vi "NI_controller_PVC.VI"(5 "Initialize":bool=TRUE, 6 "Z (mm)":dbl, 7 "Motion System":u16(ring)=3 items=["MM3000", "WMC Servo", "RRI Rot", "RRI SMAC", "Aero NI", "RRI LinInd"], 8 "error in":errorcluster, 9 "Y (mm)":dbl, 10 "X (mm)":dbl, 11 "Motion ID":T1=1 min=1 max=32 step=1) -> (0 "error out":errorcluster)   [LabVIEW 2022 SP3]
uses:
  <vilib>/Motion/FlexMotion/CustomControls/CustomControls.llb/AxisOrVectorSpace To Configure.flx
  <vilib>/Motion/FlexMotion/FunctionsVIs/StartStopMotion.llb/Start Motion (8 axes).flx
panel:
  # "X Axis"
  # "Y Axis"
  # "Z Axis"
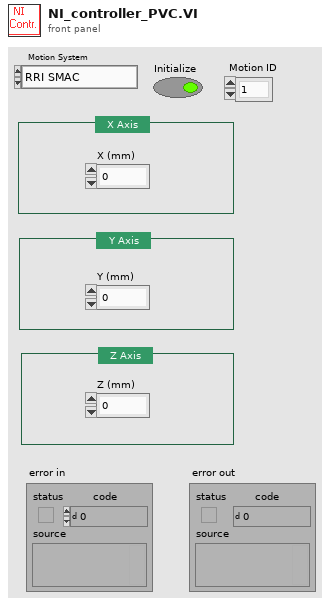
[diagram p1: front panel]
types:
  T1 = typedef "Board Id" = u8
  T2 = typedef "AxisOrVectorSpace To Configure.flx" = u16
  T3 = enum16{"Absolute Position", "Relative Position", "Velocity", "Relative to Cap Pos", "Modulus Position", "Absolute Contouring", "Relative Contouring"}
  T4 = typedef "Bd Id Out" = u8
  T5 = typedef "Resource Out (Enum).flx" = u16
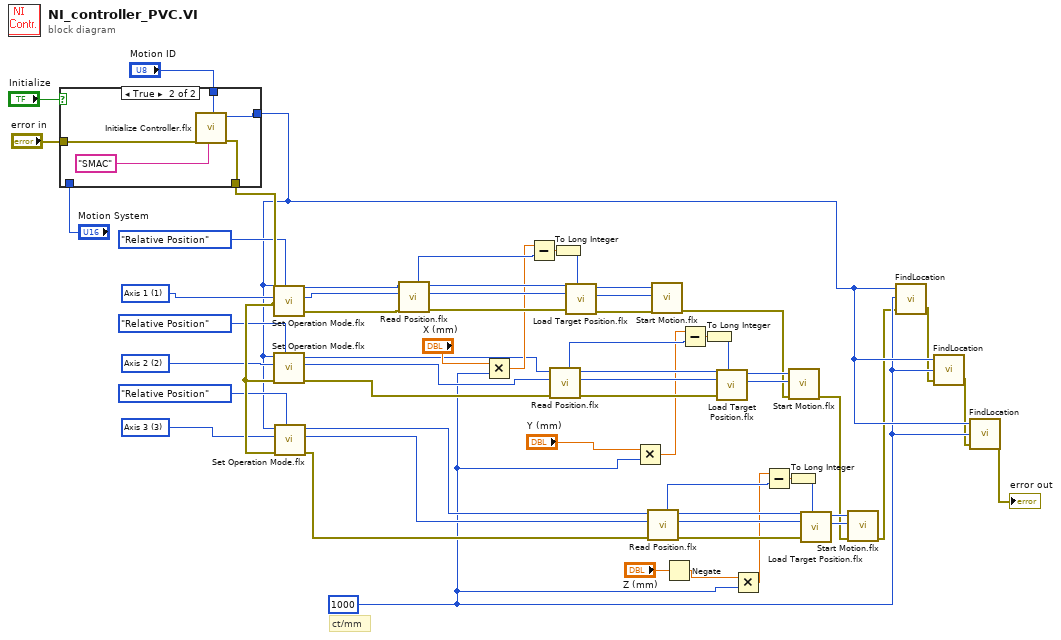
[diagram p0: block diagram]
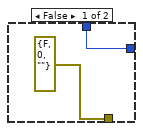
[diagram p2: hidden frame]
diagram:
  w9 = 1000 ("y")
  w49 = T2 3 items=["Axis 1"=1, "Axis 2"=2, "Axis 3"=3, "Axis 4"=4, "Axis 5"=5, "Axis 6"=6, "Vector Space 1"=17, "Vector Space 2"=18, "Vector Space 3"=19] ("Axis or Vector Space")
  w48 = T2 2 items=["Axis 1"=1, "Axis 2"=2, "Axis 3"=3, "Axis 4"=4, "Axis 5"=5, "Axis 6"=6, "Vector Space 1"=17, "Vector Space 2"=18, "Vector Space 3"=19] ("Axis or Vector Space")
  w53 = T2 1 items=["Axis 1"=1, "Axis 2"=2, "Axis 3"=3, "Axis 4"=4, "Axis 5"=5, "Axis 6"=6, "Vector Space 1"=17, "Vector Space 2"=18, "Vector Space 3"=19] ("Axis or Vector Space")
  # "ct/mm"
  n1 = case shown="True" "Initialize" {
    tunnel: [w62 w67] -> w10
    tunnel: [errorcluster {"status"=FALSE, "code"=0, "source"=""} ("error out") w66] -> w60
    tunnel: "Motion ID" -> [w62 w65]
    tunnel: "Motion System" -> [_ _]
    tunnel: "error in" -> [_ w63]
    frame False {
    }
    frame True {
      n2 = call <vilib>:"Initialize Controller.flx"("Settings Name"="SMAC", "error in (no error)"=w63, "Board ID"=w65) -> ("error out"=w66:errorcluster, "Bd ID Out"=w67:T4)  [unwired: 5 out]
    }
  }
  n3 = call <vilib>:"Set Operation Mode.flx"("Position Mode (Absolute)"=T3."Relative Position", "error in (no error)"=w60, "Axis or Vector Space"=w53, "Board ID"=w10) -> ("error out"=w55:errorcluster, "Resource Output"=w52:T5, "Bd ID Out"=w56:T4)  [unwired: 2 out]
  n4 = call <vilib>:"Set Operation Mode.flx"("Position Mode (Absolute)"=T3."Relative Position", "error in (no error)"=w60, "Axis or Vector Space"=w48, "Board ID"=w10) -> ("error out"=w14:errorcluster, "Resource Output"=w15:T5, "Bd ID Out"=w16:T4)  [unwired: 2 out]
  n5 = call <vilib>:"Set Operation Mode.flx"("Position Mode (Absolute)"=T3."Relative Position", "error in (no error)"=w60, "Axis or Vector Space"=w49, "Board ID"=w10) -> ("error out"=w13:errorcluster, "Resource Output"=w12:T5, "Bd ID Out"=w11:T4)  [unwired: 2 out]
  n6 = call <vilib>:"Read Position.flx"("error in (no error)"=w55, "Axis"=w52, "Board ID"=w56) -> ("error out"=w45:errorcluster, "Resource Output"=w46:T5, "Bd ID Out"=w47:T4, "Position"=w44:i32)  [unwired: 3 out]
  n7 = Multiply(x="X (mm)", y=w9) -> (x*y=w43:dbl)
  n8 = Subtract(x=w43, y=w44) -> (x-y=w42:dbl)
  n9 = call <vilib>:"Read Position.flx"("error in (no error)"=w14, "Axis"=w15, "Board ID"=w16) -> ("error out"=w34:errorcluster, "Resource Output"=w35:T5, "Bd ID Out"=w36:T4, "Position"=w33:i32)  [unwired: 3 out]
  n10 = To Long Integer(number=w42) -> (32bit integer=w41:i32)
  n11 = call <vilib>:"Load Target Position.flx"("Target Position (0)"=w41, "error in (no error)"=w45, "Axis"=w46, "Board ID"=w47) -> ("error out"=w38:errorcluster, "Resource Output"=w39:T5, "Bd ID Out"=w40:T4)  [unwired: 3 out]
  n12 = Multiply(x="Y (mm)", y=w9) -> (x*y=w32:dbl)
  n13 = call <vilib>:"Read Position.flx"("error in (no error)"=w13, "Axis"=w12, "Board ID"=w11) -> ("error out"=w24:errorcluster, "Resource Output"=w25:T5, "Bd ID Out"=w26:T4, "Position"=w23:i32)  [unwired: 3 out]
  n14 = call-poly <vilib>:"Start Motion.flx"("error in (no error)"=w38, "Axis or Vector Space"=w39, "Board ID"=w40) -> ("error out"=w8:errorcluster)  [unwired: 1 in, 4 out]
  n15 = Negate(x="Z (mm)") -> (-x=w1:dbl)
  n16 = Subtract(x=w32, y=w33) -> (x-y=w31:dbl)
  n17 = To Long Integer(number=w31) -> (32bit integer=w30:i32)
  n18 = call <vilib>:"Load Target Position.flx"("Target Position (0)"=w30, "error in (no error)"=w34, "Axis"=w35, "Board ID"=w36) -> ("Resource Output"=w28:T5, "Bd ID Out"=w29:T4)  [unwired: 4 out]
  n19 = Multiply(x=w1, y=w9) -> (x*y=w22:dbl)
  n20 = Subtract(x=w22, y=w23) -> (x-y=w21:dbl)
  n21 = To Long Integer(number=w21) -> (32bit integer=w20:i32)
  n22 = call-poly <vilib>:"Start Motion.flx"("error in (no error)"=w8, "Axis or Vector Space"=w28, "Board ID"=w29) -> ("error out"=w7:errorcluster)  [unwired: 1 in, 4 out]
  n23 = call <vilib>:"Load Target Position.flx"("Target Position (0)"=w20, "error in (no error)"=w24, "Axis"=w25, "Board ID"=w26) -> ("Resource Output"=w18:T5, "Bd ID Out"=w19:T4)  [unwired: 4 out]
  n24 = call-poly <vilib>:"Start Motion.flx"("error in (no error)"=w7, "Axis or Vector Space"=w18, "Board ID"=w19) -> ("error out"=w6:errorcluster)  [unwired: 1 in, 4 out]
  n25 = call "FindLocation.vi"("error in (no error)"=w6, "ct/mm"=w9, "Board ID"=w10) -> ("error out"=w5:errorcluster)  [unwired: 1 out]
  n26 = call "FindLocation.vi"("error in (no error)"=w5, "ct/mm"=w9, "Board ID"=w10) -> ("error out"=w4:errorcluster)  [unwired: 1 out]
  n27 = call "FindLocation.vi"("error in (no error)"=w4, "ct/mm"=w9, "Board ID"=w10) -> ("error out"=→"error out":errorcluster)  [unwired: 1 out]
